vi "探头数据读取.vi"(11 "编号":string) -> ()   [LabVIEW 2016, in "斯坦道多参数.lvlib"]
panel:
  out "日期/时间字符串 2":string
  out "日期/时间字符串":string
  out "运行状态":u16(ring) items=["空闲", "水样测试", "标样核查"]
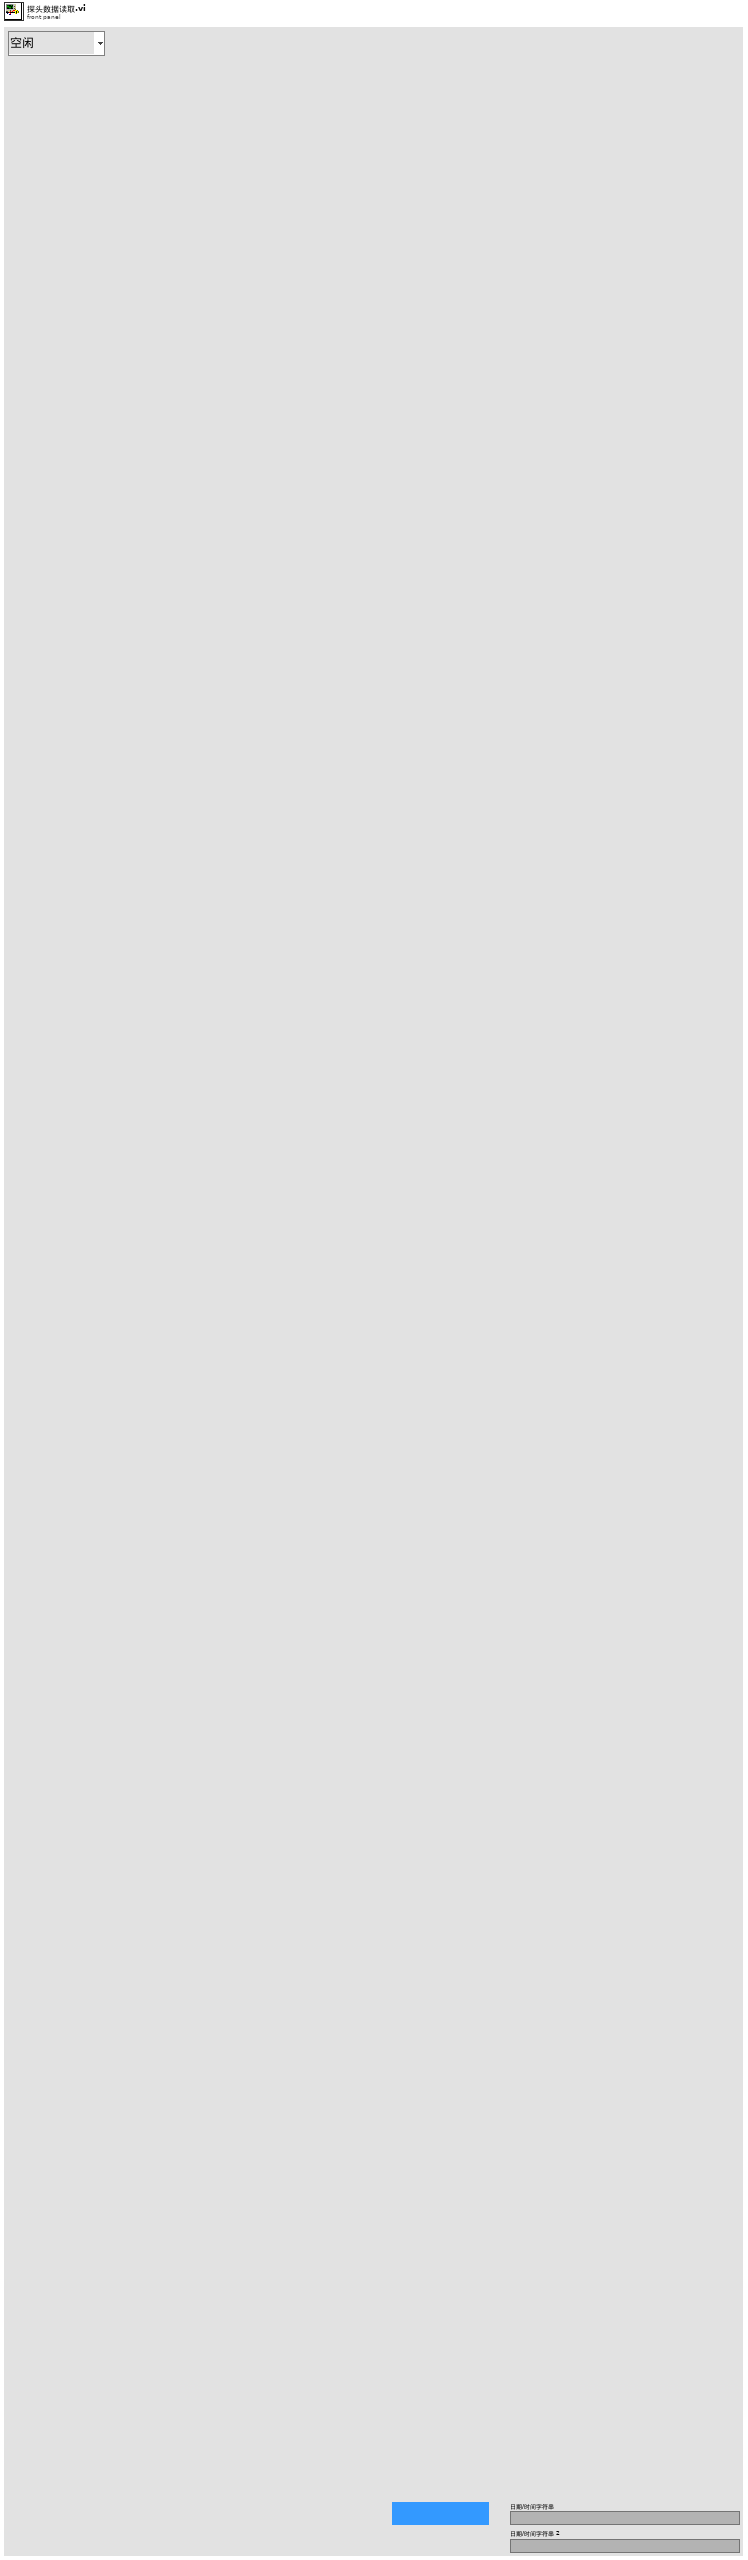
[diagram p1: front panel]
types:
  T1 = typedef "斯坦道多参数.lvlib/通知队列类型.ctl" = enum16{"pH", "DO", "DO2", "Cond", "Turb", "ORP", "叶绿素a", "藻密度", "COD"}
  T2 = cluster{"温度测量值":sgl, "测量值":sgl, "温度偏移修正值":sgl, "信号值":sgl, "数据标识":string}
  T3 = cluster{"温度测量值":sgl, "DO%":sgl, "DOmg/L":sgl, "温度偏移修正值":sgl, "数据标识mg/L":string, "数据标识%":string}
  T4 = cluster{"水温 (℃)":cluster{"量程下限":dbl, "量程上限":dbl}, "DO (mg/L)":cluster{"量程下限":dbl, "量程上限":dbl}, "DO (%)":cluster{"量程下限":dbl, "量程上限":dbl}, "pH":cluster{"量程下限":dbl, "量程上限":dbl}, "电导率 (μS/cm)":cluster{"量程下限":dbl, "量程上限":dbl}, "盐度":cluster{"量程下限":dbl, "量程上限":dbl}, "浊度 (NTU)":cluster{"量程下限":dbl, "量程上限":dbl}, "叶绿素a (μg/L)":cluster{"量程下限":dbl, "量程上限":dbl}, "藻密度 (cells/mL)":cluster{"量程下限":dbl, "量程上限":dbl}, "ORP (mV)":cluster{"量程下限":dbl, "量程上限":dbl}}
  T5 = cluster{"CH":u16, "监测值":dbl, "信号值":sgl, "数据标识":string}
  T6 = cluster{"pH探头选择":u16, "DO探头选择":u16, "电导率探头选择":u16, "浊度探头选择":u16, "叶绿素a探头选择":u16, "蓝绿藻探头选择":u16, "orp探头选择":u16, "COD探头选择":u16, "DO2探头选择":u16}
  T7 = cluster{"电极状态标志":u16, "电极型号标志":u16, "酸碱度测量值":sgl, "温度测量值":sgl, "酸碱度信号值":sgl, "温度信号值":sgl, "酸碱度偏移修正值":sgl, "温度偏移修正值":sgl, "手动温度补偿值":sgl, "酸碱度电极零点":sgl, "酸碱度电极斜率":sgl, "第1点标准值记录":sgl, "第1点信号值记录":sgl, "第1点温度值记录":sgl, "第2点标准值记录":sgl, "第2点信号值记录":sgl, "第2点温度值记录":sgl, "命令滤波设定":u16, "温度模式":enum16{"ATC", "MTC"}, "生产批次":u16, "电极序号":u16, "串口地址":u16, "串口波特率":enum16{"9600", "19200", "115200"}, "串口校验位":enum16{"NONE", "ODD", "EVEN"}, "串口停止位":enum16{"1bit", "2bit"}, "第一点标准值":sgl, "第二点标准值":sgl}
  T8 = cluster{"报警码":u16, "pH数值":sgl, "0X0003_NC":sgl, "温度数据":sgl, "pH原始信号 mv":sgl, "0X0009_NC":string, "产品名称":string, "序列号":string, "硬件版本":string, "软件版本":string, "通讯地址":u16, "波特率":u16, "设备类型":u16, "0X0026_NC":string, "第一点原始数据":sgl, "第一点校准数据":sgl, "第二点原始数据":sgl, "第二点校准数据":sgl, "探头校准命令":u16, "温度校准参数":sgl, "温度校准命令":u16}
  T9 = cluster{"电极状态标志":u16, "电极型号标志":u16, "电导率测量值":sgl, "温度测量值":sgl, "电导率信号值":sgl, "温度信号值":sgl, "温度补偿系数":sgl, "电导率偏移修正值":sgl, "温度偏移修正值":sgl, "手动温度补偿值":sgl, "电导率电极零点":sgl, "电导率电极斜率":sgl, "命令滤波设定":u16, "温度模式":enum16{"ATC", "MTC"}, "生产批次":u16, "电极序号":u16, "串口地址":u16, "串口波特率":enum16{"9600", "19200", "115200"}, "串口校验位":enum16{"NONE", "ODD", "EVEN"}, "串口停止位":enum16{"1bit", "2bit"}, "第一点标准值":sgl, "第二点标准值":sgl}
  T10 = cluster{"报警码":u16, "电导率数据（uS/cm）":sgl, "0x0003 NC":sgl, "温度数据":sgl, "电导率原始信号电阻":sgl, "当前量程":u16, "温度补偿系数":sgl, "0X0009_NC":string, "产品名称":string, "序列号":string, "硬件版本":string, "软件版本":string, "通讯地址":u16, "波特率":u16, "设备类型":u16, "0X0026_NC":string, "第一点原始数据":sgl, "第一点校准数据":sgl, "0X0035_NC":sgl, "0X0037_NC":sgl, "探头校准命令":u16, "温度校准参数":sgl, "温度校准命令":u16}
  T11 = cluster{"电极状态标志":u16, "电极型号标志":u16, "溶解氧测量值":sgl, "温度测量值":sgl, "溶解氧饱和度值":sgl, "盐度补偿值":sgl, "大气压补偿值":sgl, "溶解氧偏移修正值":sgl, "温度偏移修正值":sgl, "手动温度补偿值":sgl, "溶解氧电极零点":sgl, "溶解氧电极斜率":sgl, "第1点标准值记录":sgl, "第1点信号值记录":sgl, "第1点温度值记录":sgl, "第2点标准值记录":sgl, "第2点信号值记录":sgl, "第2点温度值记录":sgl, "命令滤波设定":u16, "温度模式":enum16{"ATC", "MTC"}, "生产批次":u16, "电极序号":u16, "串口地址":u16, "串口波特率":enum16{"9600", "19200", "115200"}, "串口校验位":enum16{"NONE", "ODD", "EVEN"}, "串口停止位":enum16{"1bit", "2bit"}, "第一点标准值":sgl, "第二点标准值":sgl}
  T12 = cluster{"报警码":u16, "溶解氧数值（mg/L）":sgl, "溶解氧数据（%）":sgl, "温度数据":sgl, "溶解氧原始信号 nA":sgl, "大气压力":sgl, "盐度":sgl, "0X0009_NC":string, "产品名称":string, "序列号":string, "硬件版本":string, "软件版本":string, "通讯地址":u16, "波特率":u16, "设备类型":u16, "0X0026_NC":string, "第一点原始数据":sgl, "0X0033 NC":sgl, "第二点原始数据":sgl, "0X0037 NC":sgl, "探头校准命令":u16, "温度校准参数":sgl, "温度校准命令":u16}
  T13 = cluster{"电极状态标志":u16, "电极型号标志":u16, "浊度测量值":sgl, "温度测量值":sgl, "浊度信号值":sgl, "浊度偏移修正值":sgl, "温度偏移修正值":sgl, "手动温度补偿值":sgl, "浊度电极零点":sgl, "浊度电极斜率":sgl, "清洁周期":u16, "命令滤波设定":u16, "温度模式":enum16{"ATC", "MTC"}, "生产批次":u16, "电极序号":u16, "串口地址":u16, "串口波特率":enum16{"9600", "19200", "115200"}, "串口校验位":enum16{"NONE", "ODD", "EVEN"}, "串口停止位":enum16{"1bit", "2bit"}, "第一点标准值":sgl, "第二点标准值":sgl, "第三点标准值":sgl}
  T14 = cluster{"报警码":u16, "浊度数值 NTU":sgl, "温度数据":sgl, "原始光强数值":u16, "量程":u16, "平均次数":u16, "清扫模式":u16, "清扫次数":u16, "清扫间隔分钟":u16, "0X000B_NC":string, "产品名称":string, "序列号":string, "硬件版本":string, "软件版本":string, "通讯地址":u16, "波特率":u16, "设备类型":u16, "0X0026_NC":string, "校准量程":u16, "第一点原始光强":u16, "第一点校准数据":sgl, "第二点原始光强":u16, "第二点校准数据":sgl, "第三点原始光强":u16, "第三点校准数据":sgl, "探头校准命令":u16, "温度校准参数":sgl, "温度校准命令":u16}
  T15 = cluster{"电极状态标志":u16, "电极型号标志":u16, "测量值":sgl, "温度测量值":sgl, "信号值":sgl, "温度信号值":sgl, "000AH_NC":sgl, "偏移修正值":sgl, "温度偏移修正值":sgl, "手动温度补偿值":sgl, "命令滤波设定":u16, "温度模式":enum16{"ATC", "MTC"}, "生产批次":u16, "传感器序号":u16, "串口地址":u16, "串口波特率":enum16{"9600", "19200", "115200"}, "串口校验位":enum16{"NONE", "ODD", "EVEN"}, "串口停止位":enum16{"1bit", "2bit"}}
  T16 = cluster{"报警码":u16, "叶绿素a":sgl, "温度数据":sgl, "原始光强数值":u16, "量程":u16, "平均次数":u16, "清扫模式":u16, "清扫次数":u16, "清扫间隔分钟":u16, "0X000B_NC":string, "产品名称":string, "序列号":string, "硬件版本":string, "软件版本":string, "通讯地址":u16, "波特率":u16, "设备类型":u16, "0X0026_NC":string, "校准量程":u16, "第一点原始光强":u16, "第一点校准数据":sgl, "第二点原始光强":u16, "第二点校准数据":sgl, "第三点原始光强":u16, "第三点校准数据":sgl, "探头校准命令":u16, "温度校准参数":sgl, "温度校准命令":u16}
  T17 = cluster{"报警码":u16, "蓝绿藻":sgl, "温度数据":sgl, "原始光强数值":u16, "0X0006_NC":u16, "平均次数":u16, "清扫模式":u16, "清扫次数":u16, "清扫间隔分钟":u16, "0X000B_NC":string, "产品名称":string, "序列号":string, "硬件版本":string, "软件版本":string, "通讯地址":u16, "波特率":u16, "设备类型":u16, "0X0026_NC":string, "0X0030_NC":u16, "第一点原始光强":u16, "第一点校准数据":sgl, "第二点原始光强":u16, "第二点校准数据":sgl, "第三点原始光强":u16, "第三点校准数据":sgl, "探头校准命令":u16, "温度校准参数":sgl, "温度校准命令":u16}
  T18 = cluster{"电极状态标志":u16, "电极型号标志":u16, "COD测量值":sgl, "浊度测量值":sgl, "COD信号值":sgl, "浊度信号值":sgl, "温度测量值":sgl, "COD偏移修正值":sgl, "浊度偏移修正值":sgl, "COD水样校正值":sgl, "温度偏移修正值":sgl, "COD零点系数":sgl, "COD斜率系数":sgl, "浊度零点系数":sgl, "浊度斜率系数":sgl, "COD测值K值":sgl, "浊度测值K值":sgl, "浊度补偿COD系数值":sgl, "COD温度补偿系数值 ":sgl, "测量周期":u16, "清洗周期":u16, "命令寄存器":u16, "数字滤波设定":u16, "温度模式":enum16{"AUTO", "OFF"}, "生产批次":u16, "电极序号":u16, "串口地址":u16, "串口波特率":enum16{"9600", "19200", "115200"}, "串口校验位":enum16{"NONE", "ODD", "EVEN"}, "串口停止位":enum16{"1bit", "2bit"}, "第一点校正指令":u16, "第一点标准值":sgl, "第二点校正指令":u16, "第二点标准值":sgl, "第三点校正指令":u16, "第三点标准值":sgl, "COD吸光度":sgl, "浊度吸光度":sgl, "温度信号值":sgl}
  T19 = cluster{"ph":bool, "DO":bool, "Cond":bool, "Turb":bool, "叶绿素a":bool, "藻密度":bool, "ORP":bool, "COD":bool, "DO2":bool}
  T20 = cluster{"ph":bool, "DO":bool, "Cond":bool, "Turb":bool, "叶绿素a":bool, "藻密度":bool, "ORP":bool, "cod":bool, "DO2":bool}
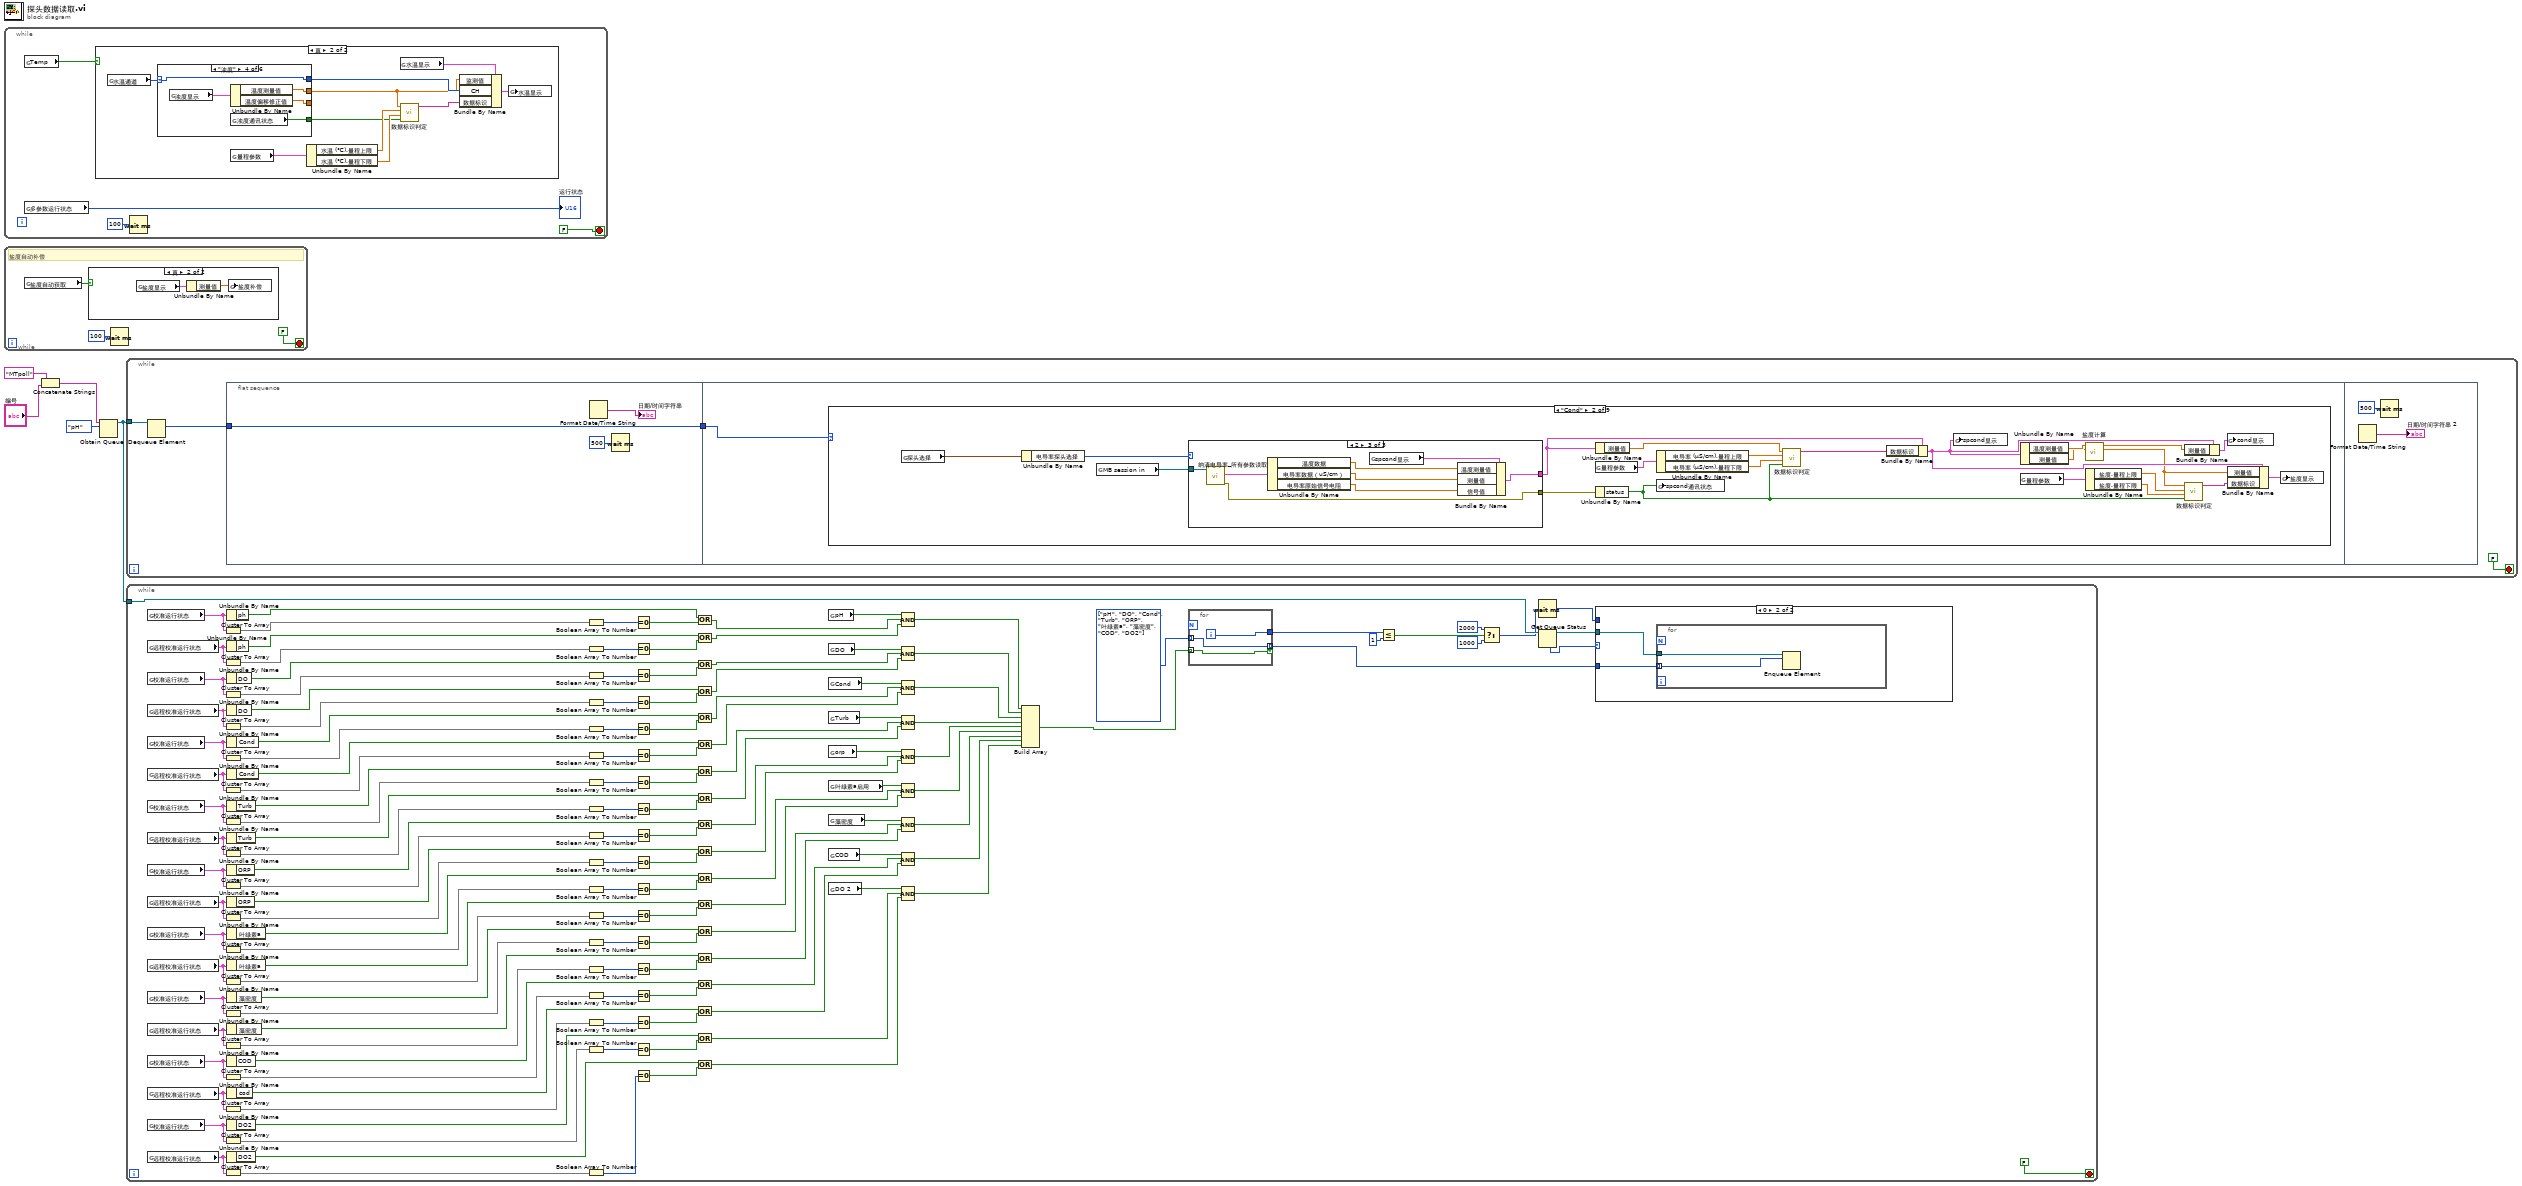
[diagram p0: block diagram]
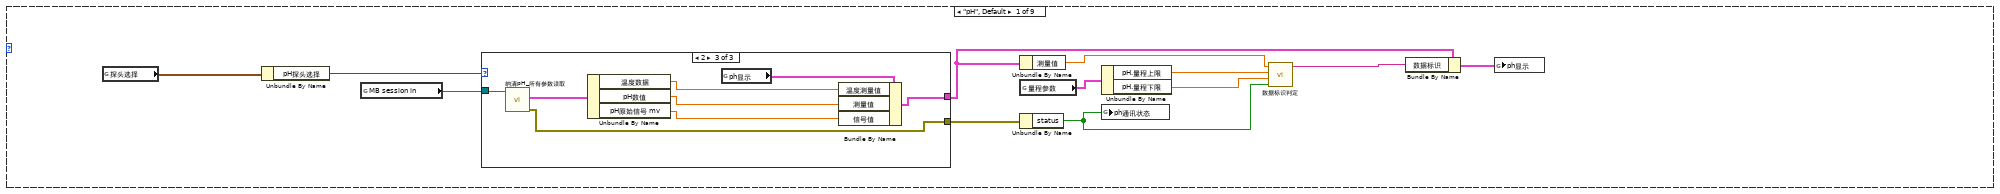
[diagram p3: hidden frame]
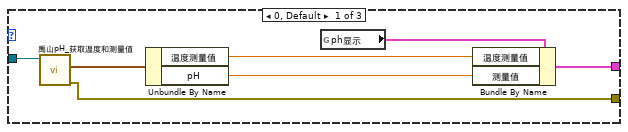
[diagram p4: hidden frame]
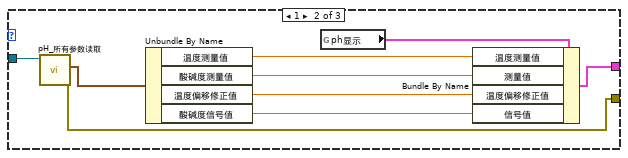
[diagram p5: hidden frame]
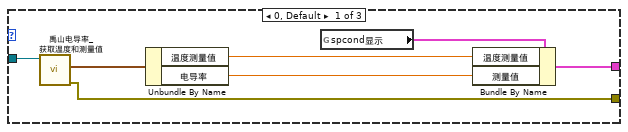
[diagram p6: hidden frame]
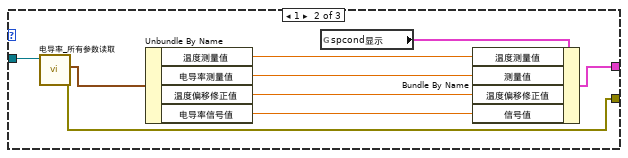
[diagram p7: hidden frame]
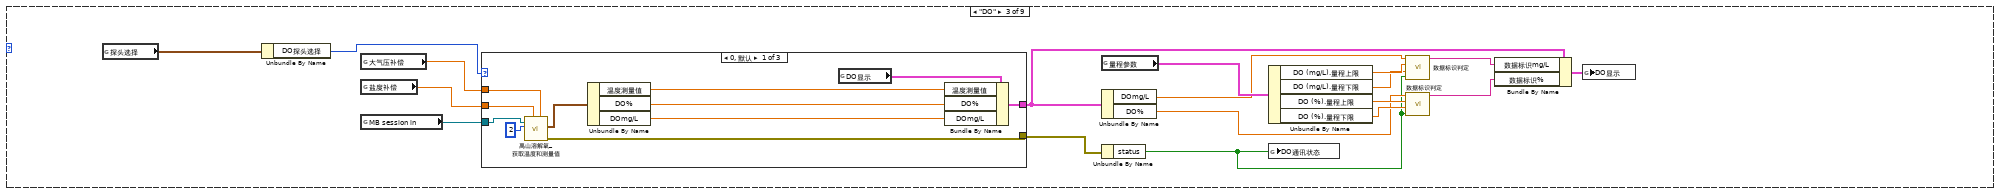
[diagram p8: hidden frame]
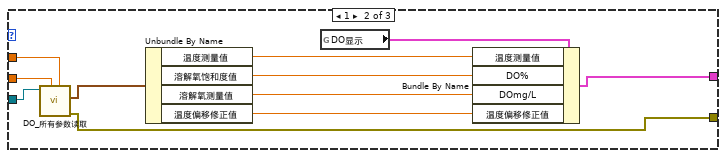
[diagram p9: hidden frame]
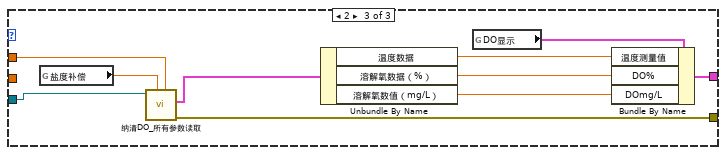
[diagram p10: hidden frame]
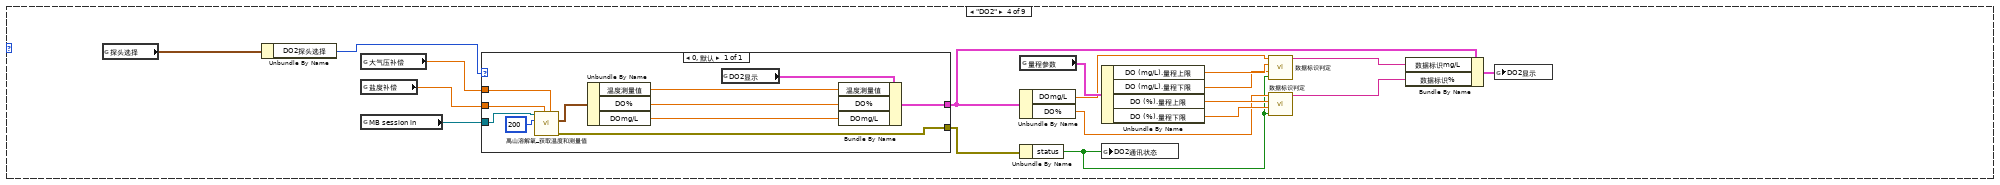
[diagram p11: hidden frame]
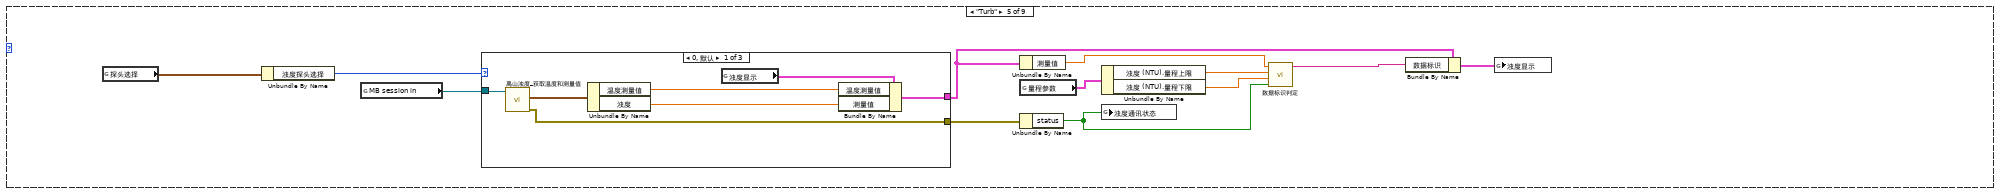
[diagram p12: hidden frame]
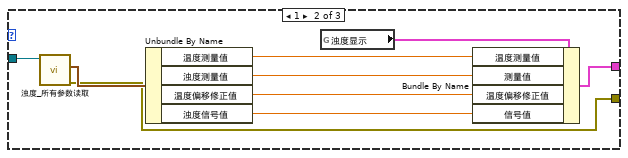
[diagram p13: hidden frame]
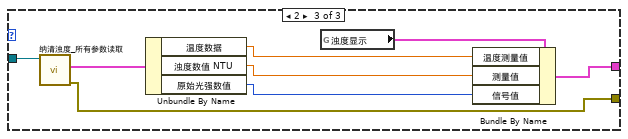
[diagram p14: hidden frame]
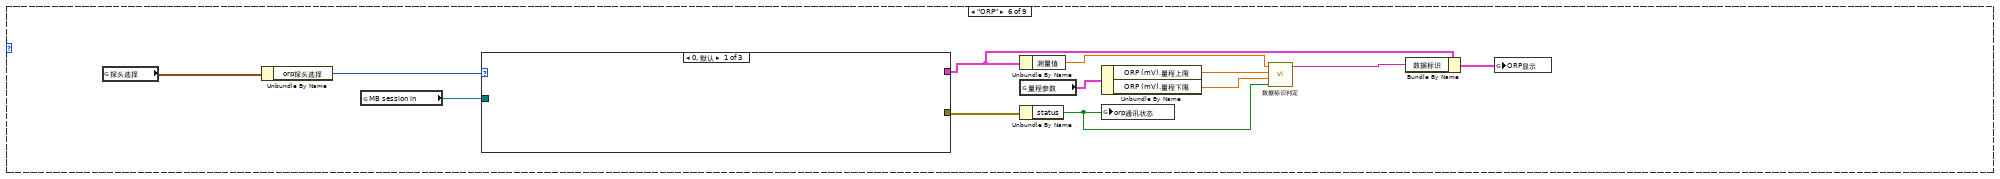
[diagram p15: hidden frame]
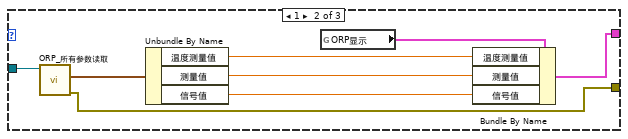
[diagram p16: hidden frame]
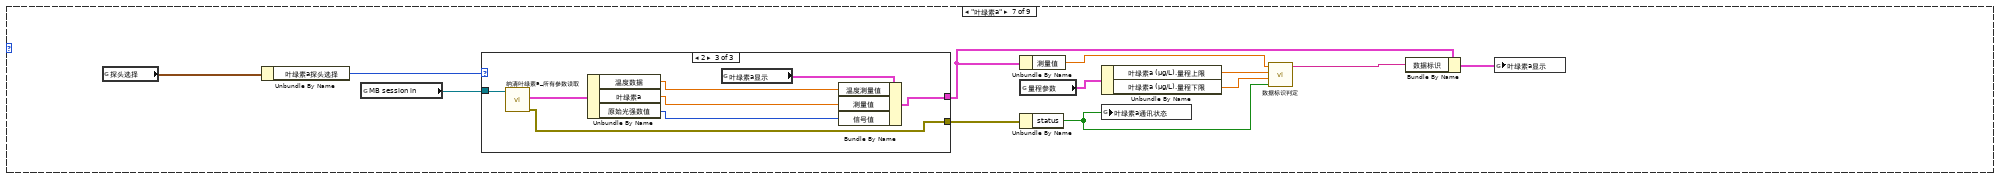
[diagram p18: hidden frame]
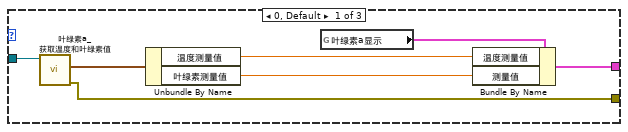
[diagram p19: hidden frame]
diagram:
  n1 = while {
    stop <- FALSE stop-if-true
    n2 = global read "断电保存变量.vi" "Temp"() -> (w7:bool)
    n3 = global read "多参数全局变量.vi" "多参数运行状态"() -> (→"运行状态":u16)
    n4 = case shown="真" w7 {
      frame False {
      }
      frame True {
        n5 = global read "断电保存变量.vi" "水温通道"() -> (w19:enum16{"pH", "DO", "浊度", "电导率", "叶绿素a", "藻密度"})
        n6 = case shown="\"浊度\"" w19 {
          selector: w19 -> [w24 w29 w34 w39 w44 w49]
          tunnel: [w24 w29 w34 w39 w44 w49] -> w18
          tunnel: [w22 w26 w31 w36 w41 w46] -> _
          tunnel: [w23 w27 w32 w37 w42 w47] -> w12
          tunnel: [w20 w25 w30 w35 w40 w45] -> w10
          frame "pH", Default {
            n7 = global read "多参数全局变量.vi" "ph显示"() -> (w21:T2)
            n8 = Unbundle By Name(w21) -> ("温度测量值"=w23:sgl, "温度偏移修正值"=w22:sgl)
            n9 = global read "多参数全局变量.vi" "ph通讯状态"() -> (w20:bool)
          }
          frame "电导率" {
            n10 = global read "多参数全局变量.vi" "spcond显示"() -> (w28:T2)
            n11 = Unbundle By Name(w28) -> ("温度测量值"=w27:sgl, "温度偏移修正值"=w26:sgl)
            n12 = global read "多参数全局变量.vi" "spcond通讯状态"() -> (w25:bool)
          }
          frame "DO" {
            n13 = global read "多参数全局变量.vi" "DO显示"() -> (w33:T3)
            n14 = Unbundle By Name(w33) -> ("温度测量值"=w32:sgl, "温度偏移修正值"=w31:sgl)
            n15 = global read "多参数全局变量.vi" "DO通讯状态"() -> (w30:bool)
          }
          frame "浊度" {
            n16 = global read "多参数全局变量.vi" "浊度显示"() -> (w38:T2)
            n17 = Unbundle By Name(w38) -> ("温度测量值"=w37:sgl, "温度偏移修正值"=w36:sgl)
            n18 = global read "多参数全局变量.vi" "浊度通讯状态"() -> (w35:bool)
          }
          frame "叶绿素a" {
            n19 = global read "多参数全局变量.vi" "叶绿素a显示"() -> (w43:T2)
            n20 = Unbundle By Name(w43) -> ("温度测量值"=w42:sgl, "温度偏移修正值"=w41:sgl)
            n21 = global read "多参数全局变量.vi" "叶绿素a通讯状态"() -> (w40:bool)
          }
          frame "藻密度" {
            n22 = global read "多参数全局变量.vi" "藻密度显示"() -> (w48:T2)
            n23 = Unbundle By Name(w48) -> ("温度测量值"=w47:sgl, "温度偏移修正值"=w46:sgl)
            n24 = global read "多参数全局变量.vi" "藻密度通讯状态"() -> (w45:bool)
          }
        }
        n25 = global read "断电保存变量.vi" "量程参数"() -> (w15:T4)
        n26 = Unbundle By Name(w15) -> ("水温 (℃).量程上限"=w13:dbl, "水温 (℃).量程下限"=w14:dbl)
        n27 = global read "多参数全局变量.vi" "水温显示"() -> (w16:T5)
        n28 = call "数据标识判定.vi"("通讯故障"=w10, "量程下限"=w14, "量程上限"=w13, "测量值"=w12) -> ("数据标识"=w11:string)  [unwired: 7 in]
        n29 = Bundle By Name(cluster=w16, "监测值"=w12, "CH"=w18, "数据标识"=w11) -> (w17:T5)
        n30 = global write "多参数全局变量.vi" "水温显示"(w17) -> ()
      }
    }
    n31 = Wait (ms)(milliseconds to wait=u32 100 ("等待时间（毫秒）")) -> ()  [unwired: 1 out]
  }
  n32 = while {
    stop <- FALSE stop-if-true
    # "盐度自动补偿"
    n33 = global read "断电保存变量.vi" "盐度自动获取"() -> (w51:bool)
    n34 = case shown="真" w51 {
      frame False {
      }
      frame True {
        n35 = global read "多参数全局变量.vi" "盐度显示"() -> (w54:T2)
        n36 = Unbundle By Name(w54) -> ("测量值"=w53:sgl)
        n37 = global write "断电保存变量.vi" "盐度补偿"(w53) -> ()
      }
    }
    n38 = Wait (ms)(milliseconds to wait=u32 100 ("等待时间（毫秒）")) -> ()  [unwired: 1 out]
  }
  n39 = Concatenate Strings("MTpoll" ("名称（未命名）"), "编号") -> (w3:string)
  n40 = Obtain Queue(name (unnamed)=w3, element data type=通知队列类型."pH" ("枚举")) -> (queue out=w1:refnum<queue>)  [unwired: 3 in, 2 out]
  n41 = while {
    tunnel: w1 -> [w58]
    stop <- FALSE stop-if-true
    n42 = Dequeue Element(queue=w58) -> (element=w57:T1)  [unwired: 2 in, 3 out]
    n43 = flat-sequence {
      tunnel: w57 -> [w61]
      tunnel: [w61] -> w55
      tunnel: w55 -> [w62]
      frame #0 {
        n44 = Format Date/Time String() -> (date/time string=→"日期/时间字符串":string)  [unwired: 3 in]
        n45 = Wait (ms)(milliseconds to wait=u32 500 ("等待时间（毫秒）")) -> ()  [unwired: 1 out]
      }
      frame #1 {
        n46 = case shown="\"Cond\"" w62 {
          frame "pH", Default {
            n47 = global read "断电保存变量.vi" "探头选择"() -> (w74:T6)
            n48 = Unbundle By Name(w74) -> ("pH探头选择"=w73:u16)
            n49 = global read "多参数全局变量.vi" "MB session in"() -> (w72:refnum<class "MB_Master.lvclass">)
            n50 = case shown="2" w73 {
              tunnel: w72 -> [w81 w90 w96]
              tunnel: [w80 w89 w94] -> w71
              tunnel: [w78 w86 w97] -> w70
              frame 0, Default {
                n51 = call "禹山pH_获取温度和测量值.vi"("MB session in"=w81) -> ("error out"=w80:errorcluster, "输出值"=w77:cluster{"温度测量值":sgl, "ORP":sgl, "pH":sgl})  [unwired: 8 in, 1 out]
                n52 = Unbundle By Name(w77) -> ("温度测量值"=w76:sgl, "pH"=w75:sgl)
                n53 = global read "多参数全局变量.vi" "ph显示"() -> (w79:T2)
                n54 = Bundle By Name(cluster=w79, "温度测量值"=w76, "测量值"=w75) -> (w78:T2)
              }
              frame 1 {
                n55 = call "pH_所有参数读取.vi"("MB session in"=w90) -> ("error out"=w89:errorcluster, "输出值"=w88:T7)  [unwired: 8 in, 1 out]
                n56 = Unbundle By Name(w88) -> ("温度测量值"=w83:sgl, "酸碱度测量值"=w84:sgl, "温度偏移修正值"=w85:sgl, "酸碱度信号值"=w82:sgl)
                n57 = global read "多参数全局变量.vi" "ph显示"() -> (w87:T2)
                n58 = Bundle By Name(cluster=w87, "温度测量值"=w83, "测量值"=w84, "温度偏移修正值"=w85, "信号值"=w82) -> (w86:T2)
              }
              frame 2 {
                n59 = call "纳清pH_所有参数读取.vi"("MB session in"=w96) -> ("error out"=w94:errorcluster, "输出值"=w95:T8)  [unwired: 8 in, 1 out]
                n60 = Unbundle By Name(w95) -> ("温度数据"=w93:sgl, "pH数值"=w92:sgl, "pH原始信号 mv"=w91:sgl)
                n61 = global read "多参数全局变量.vi" "ph显示"() -> (w98:T2)
                n62 = Bundle By Name(cluster=w98, "温度测量值"=w93, "测量值"=w92, "信号值"=w91) -> (w97:T2)
              }
            }
            n63 = Unbundle By Name(w70) -> ("测量值"=w68:sgl)
            n64 = global read "断电保存变量.vi" "量程参数"() -> (w69:T4)
            n65 = Unbundle By Name(w71) -> ("status"=w65:bool)
            n66 = Unbundle By Name(w69) -> ("pH.量程上限"=w67:dbl, "pH.量程下限"=w66:dbl)
            n67 = global write "多参数全局变量.vi" "ph通讯状态"(w65) -> ()
            n68 = call "数据标识判定.vi"("通讯故障"=w65, "量程下限"=w66, "量程上限"=w67, "测量值"=w68) -> ("数据标识"=w63:string)  [unwired: 7 in]
            n69 = Bundle By Name(cluster=w70, "数据标识"=w63) -> (w64:T2)
            n70 = global write "多参数全局变量.vi" "ph显示"(w64) -> ()
          }
          frame "Cond" {
            n71 = global read "断电保存变量.vi" "探头选择"() -> (w120:T6)
            n72 = Unbundle By Name(w120) -> ("电导率探头选择"=w119:u16)
            n73 = global read "多参数全局变量.vi" "MB session in"() -> (w118:refnum<class "MB_Master.lvclass">)
            n74 = case shown="2" w119 {
              tunnel: w118 -> [w127 w136 w140]
              tunnel: [w121 w134 w143] -> w113
              tunnel: [w126 w133 w138] -> w117
              frame 0, Default {
                n75 = call "禹山电导率_获取温度和测量值.vi"("MB session in"=w127) -> ("error out"=w126:errorcluster, "输出值"=w124:cluster{"温度测量值":sgl, "电导率":sgl, "错误标志":u16})  [unwired: 8 in, 1 out]
                n76 = Unbundle By Name(w124) -> ("温度测量值"=w123:sgl, "电导率"=w122:sgl)
                n77 = global read "多参数全局变量.vi" "spcond显示"() -> (w125:T2)
                n78 = Bundle By Name(cluster=w125, "温度测量值"=w123, "测量值"=w122) -> (w121:T2)
              }
              frame 1 {
                n79 = call "电导率_所有参数读取.vi"("MB session in"=w136) -> ("error out"=w133:errorcluster, "输出值"=w132:T9)  [unwired: 8 in, 1 out]
                n80 = Unbundle By Name(w132) -> ("温度测量值"=w131:sgl, "电导率测量值"=w130:sgl, "温度偏移修正值"=w129:sgl, "电导率信号值"=w128:sgl)
                n81 = global read "多参数全局变量.vi" "spcond显示"() -> (w135:T2)
                n82 = Bundle By Name(cluster=w135, "温度测量值"=w131, "测量值"=w130, "温度偏移修正值"=w129, "信号值"=w128) -> (w134:T2)
              }
              frame 2 {
                n83 = call "纳清电导率_所有参数读取.vi"("MB session in"=w140) -> ("error out"=w138:errorcluster, "输出值"=w139:T10)  [unwired: 8 in, 1 out]
                n84 = Unbundle By Name(w139) -> ("温度数据"=w142:sgl, "电导率数据（uS/cm）"=w141:sgl, "电导率原始信号电阻"=w137:sgl)
                n85 = global read "多参数全局变量.vi" "spcond显示"() -> (w144:T2)
                n86 = Bundle By Name(cluster=w144, "温度测量值"=w142, "测量值"=w141, "信号值"=w137) -> (w143:T2)
              }
            }
            n87 = Unbundle By Name(w113) -> ("测量值"=w112:sgl)
            n88 = global read "断电保存变量.vi" "量程参数"() -> (w116:T4)
            n89 = Unbundle By Name(w117) -> ("status"=w109:bool)
            n90 = Unbundle By Name(w116) -> ("电导率 (μS/cm).量程上限"=w115:dbl, "电导率 (μS/cm).量程下限"=w114:dbl)
            n91 = global write "多参数全局变量.vi" "spcond通讯状态"(w109) -> ()
            n92 = call "数据标识判定.vi"("通讯故障"=w109, "量程下限"=w114, "量程上限"=w115, "测量值"=w112) -> ("数据标识"=w110:string)  [unwired: 7 in]
            n93 = Bundle By Name(cluster=w113, "数据标识"=w110) -> (w111:T2)
            n94 = global write "多参数全局变量.vi" "spcond显示"(w111) -> ()
            n95 = Unbundle By Name(w111) -> ("温度测量值"=w108:sgl, "测量值"=w107:sgl)
            n96 = global read "断电保存变量.vi" "量程参数"() -> (w101:T4)
            n97 = call "盐度计算.vi"("spCond"=w107, "Temp"=w108) -> ("saltresult"=w100:dbl, "cond"=w106:dbl)  [unwired: 8 in]
            n98 = Unbundle By Name(w101) -> ("盐度.量程上限"=w102:dbl, "盐度.量程下限"=w103:dbl)
            n99 = Bundle By Name(cluster=w111, "测量值"=w106) -> (w105:T2)
            n100 = call "数据标识判定.vi"("通讯故障"=w109, "量程下限"=w103, "量程上限"=w102, "测量值"=w100) -> ("数据标识"=w99:string)  [unwired: 7 in]
            n101 = global write "多参数全局变量.vi" "cond显示"(w105) -> ()
            n102 = Bundle By Name(cluster=w111, "测量值"=w100, "数据标识"=w99) -> (w104:T2)
            n103 = global write "多参数全局变量.vi" "盐度显示"(w104) -> ()
          }
          frame "DO" {
            n104 = global read "断电保存变量.vi" "探头选择"() -> (w162:T6)
            n105 = Unbundle By Name(w162) -> ("DO探头选择"=w161:u16)
            n106 = global read "断电保存变量.vi" "大气压补偿"() -> (w145:dbl)
            n107 = global read "断电保存变量.vi" "盐度补偿"() -> (w146:dbl)
            n108 = global read "多参数全局变量.vi" "MB session in"() -> (w160:refnum<class "MB_Master.lvclass">)
            n109 = case shown="0, 默认" w161 {
              tunnel: w160 -> [w173 w184 w189]
              tunnel: [w171 w182 w193] -> w153
              tunnel: [w167 w177 w187] -> w159
              tunnel: w146 -> [w164 w175 _]
              tunnel: w145 -> [w163 w174 w185]
              frame 0, Default {
                n110 = call "禹山溶解氧_获取温度和测量值.vi"("大气压补偿"=w163, "盐度补偿"=w164, "salve ID"=u16 2, "MB session in"=w173) -> ("error out"=w167:errorcluster, "输出值"=w166:cluster{"温度测量值":sgl, "DO%":sgl, "DOmg/L":sgl})  [unwired: 5 in, 1 out]
                n111 = Unbundle By Name(w166) -> ("温度测量值"=w170:sgl, "DO%"=w169:sgl, "DOmg/L"=w168:sgl)
                n112 = global read "多参数全局变量.vi" "DO显示"() -> (w172:T3)
                n113 = Bundle By Name(cluster=w172, "温度测量值"=w170, "DO%"=w169, "DOmg/L"=w168) -> (w171:T3)
              }
              frame 1 {
                n114 = call "DO_所有参数读取.vi"("大气压补偿"=w174, "盐度补偿"=w175, "MB session in"=w184) -> ("error out"=w177:errorcluster, "输出值"=w181:T11)  [unwired: 6 in, 1 out]
                n115 = Unbundle By Name(w181) -> ("温度测量值"=w178:sgl, "溶解氧饱和度值"=w179:sgl, "溶解氧测量值"=w180:sgl, "温度偏移修正值"=w176:sgl)
                n116 = global read "多参数全局变量.vi" "DO显示"() -> (w183:T3)
                n117 = Bundle By Name(cluster=w183, "温度测量值"=w178, "DO%"=w179, "DOmg/L"=w180, "温度偏移修正值"=w176) -> (w182:T3)
              }
              frame 2 {
                n118 = global read "断电保存变量.vi" "盐度补偿"() -> (w186:dbl)
                n119 = call "纳清DO_所有参数读取.vi"("大气压补偿"=w185, "盐度补偿"=w186, "MB session in"=w189) -> ("error out"=w187:errorcluster, "输出值"=w188:T12)  [unwired: 6 in, 1 out]
                n120 = Unbundle By Name(w188) -> ("温度数据"=w190:sgl, "溶解氧数据（%）"=w191:sgl, "溶解氧数值（mg/L）"=w192:sgl)
                n121 = global read "多参数全局变量.vi" "DO显示"() -> (w194:T3)
                n122 = Bundle By Name(cluster=w194, "温度测量值"=w190, "DO%"=w191, "DOmg/L"=w192) -> (w193:T3)
              }
            }
            n123 = global read "断电保存变量.vi" "量程参数"() -> (w158:T4)
            n124 = Unbundle By Name(w153) -> ("DOmg/L"=w152:sgl, "DO%"=w151:sgl)
            n125 = Unbundle By Name(w159) -> ("status"=w147:bool)
            n126 = Unbundle By Name(w158) -> ("DO (mg/L).量程上限"=w157:dbl, "DO (mg/L).量程下限"=w156:dbl, "DO (%).量程上限"=w155:dbl, "DO (%).量程下限"=w154:dbl)
            n127 = global write "多参数全局变量.vi" "DO通讯状态"(w147) -> ()
            n128 = call "数据标识判定.vi"("通讯故障"=w147, "量程下限"=w156, "量程上限"=w157, "测量值"=w152) -> ("数据标识"=w149:string)  [unwired: 7 in]
            n129 = call "数据标识判定.vi"("通讯故障"=w147, "量程下限"=w154, "量程上限"=w155, "测量值"=w151) -> ("数据标识"=w148:string)  [unwired: 7 in]
            n130 = Bundle By Name(cluster=w153, "数据标识mg/L"=w149, "数据标识%"=w148) -> (w150:T3)
            n131 = global write "多参数全局变量.vi" "DO显示"(w150) -> ()
          }
          frame "DO2" {
            n132 = global read "断电保存变量.vi" "探头选择"() -> (w212:T6)
            n133 = Unbundle By Name(w212) -> ("DO2探头选择"=w211:u16)
            n134 = global read "断电保存变量.vi" "大气压补偿"() -> (w195:dbl)
            n135 = global read "断电保存变量.vi" "盐度补偿"() -> (w196:dbl)
            n136 = global read "多参数全局变量.vi" "MB session in"() -> (w210:refnum<class "MB_Master.lvclass">)
            n137 = case shown="0, 默认" w211 {
              tunnel: w210 -> [w223]
              tunnel: [w221] -> w203
              tunnel: [w217] -> w209
              tunnel: w196 -> [w214]
              tunnel: w195 -> [w213]
              frame 0, Default {
                n138 = call "禹山溶解氧_获取温度和测量值.vi"("大气压补偿"=w213, "盐度补偿"=w214, "salve ID"=u16 200, "MB session in"=w223) -> ("error out"=w217:errorcluster, "输出值"=w216:cluster{"温度测量值":sgl, "DO%":sgl, "DOmg/L":sgl})  [unwired: 5 in, 1 out]
                n139 = Unbundle By Name(w216) -> ("温度测量值"=w220:sgl, "DO%"=w219:sgl, "DOmg/L"=w218:sgl)
                n140 = global read "多参数全局变量.vi" "DO2显示"() -> (w222:T3)
                n141 = Bundle By Name(cluster=w222, "温度测量值"=w220, "DO%"=w219, "DOmg/L"=w218) -> (w221:T3)
              }
            }
            n142 = global read "断电保存变量.vi" "量程参数"() -> (w208:T4)
            n143 = Unbundle By Name(w203) -> ("DOmg/L"=w202:sgl, "DO%"=w201:sgl)
            n144 = Unbundle By Name(w209) -> ("status"=w197:bool)
            n145 = Unbundle By Name(w208) -> ("DO (mg/L).量程上限"=w207:dbl, "DO (mg/L).量程下限"=w206:dbl, "DO (%).量程上限"=w205:dbl, "DO (%).量程下限"=w204:dbl)
            n146 = global write "多参数全局变量.vi" "DO2通讯状态"(w197) -> ()
            n147 = call "数据标识判定.vi"("通讯故障"=w197, "量程下限"=w206, "量程上限"=w207, "测量值"=w202) -> ("数据标识"=w199:string)  [unwired: 7 in]
            n148 = call "数据标识判定.vi"("通讯故障"=w197, "量程下限"=w204, "量程上限"=w205, "测量值"=w201) -> ("数据标识"=w198:string)  [unwired: 7 in]
            n149 = Bundle By Name(cluster=w203, "数据标识mg/L"=w199, "数据标识%"=w198) -> (w200:T3)
            n150 = global write "多参数全局变量.vi" "DO2显示"(w200) -> ()
          }
          frame "Turb" {
            n151 = global read "断电保存变量.vi" "探头选择"() -> (w235:T6)
            n152 = Unbundle By Name(w235) -> ("浊度探头选择"=w234:u16)
            n153 = global read "多参数全局变量.vi" "MB session in"() -> (w233:refnum<class "MB_Master.lvclass">)
            n154 = case shown="0, 默认" w234 {
              tunnel: w233 -> [w242 w251 w255]
              tunnel: [w240 w246 w256] -> w227
              tunnel: [w239 w245 w254] -> w232
              frame 0, Default {
                n155 = call "禹山浊度_获取温度和测量值.vi"("MB session in"=w242) -> ("error out"=w239:errorcluster, "输出值"=w238:cluster{"温度测量值":sgl, "浊度":sgl})  [unwired: 8 in, 1 out]
                n156 = Unbundle By Name(w238) -> ("温度测量值"=w237:sgl, "浊度"=w236:sgl)
                n157 = global read "多参数全局变量.vi" "浊度显示"() -> (w241:T2)
                n158 = Bundle By Name(cluster=w241, "温度测量值"=w237, "测量值"=w236) -> (w240:T2)
              }
              frame 1 {
                n159 = call "浊度_所有参数读取.vi"("MB session in"=w251) -> ("error out"=w245:errorcluster, "输出值"=w250:T13)  [unwired: 8 in, 1 out]
                n160 = Unbundle By Name(w250) -> ("温度测量值"=w248:sgl, "浊度测量值"=w247:sgl, "温度偏移修正值"=w244:sgl, "浊度信号值"=w243:sgl)
                n161 = global read "多参数全局变量.vi" "浊度显示"() -> (w249:T2)
                n162 = Bundle By Name(cluster=w249, "温度测量值"=w248, "测量值"=w247, "温度偏移修正值"=w244, "信号值"=w243) -> (w246:T2)
              }
              frame 2 {
                n163 = call "纳清浊度_所有参数读取.vi"("MB session in"=w255) -> ("error out"=w254:errorcluster, "输出值"=w253:T14)  [unwired: 8 in, 1 out]
                n164 = Unbundle By Name(w253) -> ("温度数据"=w258:sgl, "浊度数值 NTU"=w257:sgl, "原始光强数值"=w252:u16)
                n165 = global read "多参数全局变量.vi" "浊度显示"() -> (w259:T2)
                n166 = Bundle By Name(cluster=w259, "温度测量值"=w258, "测量值"=w257, "信号值"=w252) -> (w256:T2)
              }
            }
            n167 = Unbundle By Name(w227) -> ("测量值"=w226:sgl)
            n168 = global read "断电保存变量.vi" "量程参数"() -> (w231:T4)
            n169 = Unbundle By Name(w232) -> ("status"=w228:bool)
            n170 = Unbundle By Name(w231) -> ("浊度 (NTU).量程上限"=w230:dbl, "浊度 (NTU).量程下限"=w229:dbl)
            n171 = global write "多参数全局变量.vi" "浊度通讯状态"(w228) -> ()
            n172 = call "数据标识判定.vi"("通讯故障"=w228, "量程下限"=w229, "量程上限"=w230, "测量值"=w226) -> ("数据标识"=w224:string)  [unwired: 7 in]
            n173 = Bundle By Name(cluster=w227, "数据标识"=w224) -> (w225:T2)
            n174 = global write "多参数全局变量.vi" "浊度显示"(w225) -> ()
          }
          frame "ORP" {
            n175 = global read "断电保存变量.vi" "探头选择"() -> (w271:T6)
            n176 = Unbundle By Name(w271) -> ("orp探头选择"=w270:u16)
            n177 = global read "多参数全局变量.vi" "MB session in"() -> (w269:refnum<class "MB_Master.lvclass">)
            n178 = case shown="0, 默认" w270 {
              tunnel: [_ w274 _] -> w268
              tunnel: w269 -> [_ w279 _]
              tunnel: [_ w272 _] -> w263
              frame 0, Default {
              }
              frame 1 {
                n179 = call "ORP_所有参数读取.vi"("MB session in"=w279) -> ("error out"=w274:errorcluster, "输出值"=w276:T15)  [unwired: 8 in, 1 out]
                n180 = Unbundle By Name(w276) -> ("温度测量值"=w277:sgl, "测量值"=w278:sgl, "信号值"=w273:sgl)
                n181 = global read "多参数全局变量.vi" "ORP显示"() -> (w275:T2)
                n182 = Bundle By Name(cluster=w275, "温度测量值"=w277, "测量值"=w278, "信号值"=w273) -> (w272:T2)
              }
              frame 2 {
              }
            }
            n183 = Unbundle By Name(w263) -> ("测量值"=w262:sgl)
            n184 = global read "断电保存变量.vi" "量程参数"() -> (w267:T4)
            n185 = Unbundle By Name(w268) -> ("status"=w264:bool)
            n186 = Unbundle By Name(w267) -> ("ORP (mV).量程上限"=w266:dbl, "ORP (mV).量程下限"=w265:dbl)
            n187 = global write "多参数全局变量.vi" "orp通讯状态"(w264) -> ()
            n188 = call "数据标识判定.vi"("通讯故障"=w264, "量程下限"=w265, "量程上限"=w266, "测量值"=w262) -> ("数据标识"=w260:string)  [unwired: 7 in]
            n189 = Bundle By Name(cluster=w263, "数据标识"=w260) -> (w261:T2)
            n190 = global write "多参数全局变量.vi" "ORP显示"(w261) -> ()
          }
          frame "叶绿素a" {
            n191 = global read "断电保存变量.vi" "探头选择"() -> (w291:T6)
            n192 = Unbundle By Name(w291) -> ("叶绿素a探头选择"=w290:u16)
            n193 = global read "多参数全局变量.vi" "MB session in"() -> (w289:refnum<class "MB_Master.lvclass">)
            n194 = case shown="2" w290 {
              tunnel: [w298 _ w304] -> w288
              tunnel: w289 -> [w297 _ w306]
              tunnel: [w295 _ w303] -> w284
              frame 0, Default {
                n195 = call "叶绿素a_获取温度和叶绿素值.vi"("MB session in"=w297) -> ("error out"=w298:errorcluster, "输出值"=w294:cluster{"温度测量值":sgl, "叶绿素测量值":sgl, "错误标志":u16})  [unwired: 8 in, 1 out]
                n196 = Unbundle By Name(w294) -> ("温度测量值"=w292:sgl, "叶绿素测量值"=w293:sgl)
                n197 = global read "多参数全局变量.vi" "叶绿素a显示"() -> (w296:T2)
                n198 = Bundle By Name(cluster=w296, "温度测量值"=w292, "测量值"=w293) -> (w295:T2)
              }
              frame 1 {
              }
              frame 2 {
                n199 = call "纳清叶绿素a_所有参数读取.vi"("MB session in"=w306) -> ("error out"=w304:errorcluster, "输出值"=w302:T16)  [unwired: 8 in, 1 out]
                n200 = Unbundle By Name(w302) -> ("温度数据"=w300:sgl, "叶绿素a"=w301:sgl, "原始光强数值"=w299:u16)
                n201 = global read "多参数全局变量.vi" "叶绿素a显示"() -> (w305:T2)
                n202 = Bundle By Name(cluster=w305, "温度测量值"=w300, "测量值"=w301, "信号值"=w299) -> (w303:T2)
              }
            }
            n203 = Unbundle By Name(w284) -> ("测量值"=w283:sgl)
            n204 = global read "断电保存变量.vi" "量程参数"() -> (w287:T4)
            n205 = Unbundle By Name(w288) -> ("status"=w282:bool)
            n206 = Unbundle By Name(w287) -> ("叶绿素a (μg/L).量程上限"=w286:dbl, "叶绿素a (μg/L).量程下限"=w285:dbl)
            n207 = global write "多参数全局变量.vi" "叶绿素a通讯状态"(w282) -> ()
            n208 = call "数据标识判定.vi"("通讯故障"=w282, "量程下限"=w285, "量程上限"=w286, "测量值"=w283) -> ("数据标识"=w280:string)  [unwired: 7 in]
            n209 = Bundle By Name(cluster=w284, "数据标识"=w280) -> (w281:T2)
            n210 = global write "多参数全局变量.vi" "叶绿素a显示"(w281) -> ()
          }
          frame "藻密度" {
            n211 = global read "断电保存变量.vi" "探头选择"() -> (w318:T6)
            n212 = Unbundle By Name(w318) -> ("蓝绿藻探头选择"=w317:u16)
            n213 = global read "多参数全局变量.vi" "MB session in"() -> (w316:refnum<class "MB_Master.lvclass">)
            n214 = case shown="2" w317 {
              tunnel: [_ _ w324] -> w315
              tunnel: w316 -> [_ _ w326]
              tunnel: [_ _ w323] -> w311
              frame 0, Default {
              }
              frame 1 {
              }
              frame 2 {
                n215 = call "纳清蓝绿藻_所有参数读取.vi"("MB session in"=w326) -> ("error out"=w324:errorcluster, "输出值"=w322:T17)  [unwired: 8 in, 1 out]
                n216 = Unbundle By Name(w322) -> ("温度数据"=w321:sgl, "蓝绿藻"=w320:sgl, "原始光强数值"=w319:u16)
                n217 = global read "多参数全局变量.vi" "藻密度显示"() -> (w325:T2)
                n218 = Bundle By Name(cluster=w325, "温度测量值"=w321, "测量值"=w320, "信号值"=w319) -> (w323:T2)
              }
            }
            n219 = Unbundle By Name(w311) -> ("测量值"=w310:sgl)
            n220 = global read "断电保存变量.vi" "量程参数"() -> (w314:T4)
            n221 = Unbundle By Name(w315) -> ("status"=w309:bool)
            n222 = Unbundle By Name(w314) -> ("藻密度 (cells/mL).量程上限"=w313:dbl, "藻密度 (cells/mL).量程下限"=w312:dbl)
            n223 = global write "多参数全局变量.vi" "藻密度通讯状态"(w309) -> ()
            n224 = call "数据标识判定.vi"("通讯故障"=w309, "量程下限"=w312, "量程上限"=w313, "测量值"=w310) -> ("数据标识"=w307:string)  [unwired: 7 in]
            n225 = Bundle By Name(cluster=w311, "数据标识"=w307) -> (w308:T2)
            n226 = global write "多参数全局变量.vi" "藻密度显示"(w308) -> ()
          }
          frame "COD" {
            n227 = global read "断电保存变量.vi" "探头选择"() -> (w337:T6)
            n228 = Unbundle By Name(w337) -> ("COD探头选择"=w336:u16)
            n229 = global read "多参数全局变量.vi" "MB session in"() -> (w335:refnum<class "MB_Master.lvclass">)
            n230 = case shown="1" w336 {
              tunnel: [_ w343 _] -> w334
              tunnel: w335 -> [_ w345 _]
              tunnel: [_ w342 _] -> w333
              frame 0, Default {
              }
              frame 1 {
                n231 = call "COD_所有参数读取.vi"("MB session in"=w345) -> ("error out"=w343:errorcluster, "输出值"=w341:T18)  [unwired: 8 in, 1 out]
                n232 = Unbundle By Name(w341) -> ("温度测量值"=w340:sgl, "COD测量值"=w339:sgl, "COD信号值"=w338:sgl)
                n233 = global read "多参数全局变量.vi" "COD显示"() -> (w344:T2)
                n234 = Bundle By Name(cluster=w344, "温度测量值"=w340, "测量值"=w339, "信号值"=w338) -> (w342:T2)
              }
              frame 2 {
              }
            }
            n235 = Unbundle By Name(w333) -> ("测量值"=w332:sgl)
            n236 = Unbundle By Name(w334) -> ("status"=w331:bool)
            n237 = global write "多参数全局变量.vi" "cod通讯状态"(w331) -> ()
            n238 = call "数据标识判定.vi"("通讯故障"=w331, "量程下限"=0.0, "量程上限"=1000.0, "测量值"=w332) -> ("数据标识"=w329:string)  [unwired: 7 in]
            n239 = Bundle By Name(cluster=w333, "数据标识"=w329) -> (w330:T2)
            n240 = case shown="无错误" w334 {
              tunnel: w330 -> [w346 _]
              frame No Error {
                n241 = global write "多参数全局变量.vi" "COD显示"(w346) -> ()
              }
              frame Error {
              }
            }
          }
        }
      }
      frame #2 {
        n242 = Format Date/Time String() -> (date/time string=→"日期/时间字符串 2":string)  [unwired: 3 in]
        n243 = Wait (ms)(milliseconds to wait=u32 500 ("等待时间（毫秒）")) -> ()  [unwired: 1 out]
      }
    }
  }
  n244 = while {
    tunnel: w1 -> [w488]
    stop <- FALSE stop-if-true
    w388 = T1[] [enum."pH", enum."DO", enum."Cond", enum."Turb", enum."ORP", enum."叶绿素a", enum."藻密度", enum."COD", enum."DO2"] items=["pH", "DO", "DO2", "Cond", "Turb", "ORP", "叶绿素a", "藻密度", "COD"]
    n245 = global read "多参数全局变量.vi" "校准运行状态"() -> (w474:T19)
    n246 = global read "多参数全局变量.vi" "远程校准运行状态"() -> (w485:T20)
    n247 = global read "多参数全局变量.vi" "校准运行状态"() -> (w448:T19)
    n248 = global read "多参数全局变量.vi" "远程校准运行状态"() -> (w459:T20)
    n249 = global read "多参数全局变量.vi" "校准运行状态"() -> (w473:T19)
    n250 = global read "多参数全局变量.vi" "远程校准运行状态"() -> (w462:T20)
    n251 = global read "多参数全局变量.vi" "校准运行状态"() -> (w435:T19)
    n252 = global read "多参数全局变量.vi" "远程校准运行状态"() -> (w446:T20)
    n253 = global read "多参数全局变量.vi" "校准运行状态"() -> (w422:T19)
    n254 = global read "多参数全局变量.vi" "远程校准运行状态"() -> (w433:T20)
    n255 = global read "多参数全局变量.vi" "校准运行状态"() -> (w421:T19)
    n256 = global read "多参数全局变量.vi" "远程校准运行状态"() -> (w410:T20)
    n257 = global read "多参数全局变量.vi" "校准运行状态"() -> (w396:T19)
    n258 = global read "多参数全局变量.vi" "远程校准运行状态"() -> (w407:T20)
    n259 = global read "多参数全局变量.vi" "校准运行状态"() -> (w383:T19)
    n260 = global read "多参数全局变量.vi" "远程校准运行状态"() -> (w376:T20)
    n261 = global read "多参数全局变量.vi" "校准运行状态"() -> (w369:T19)
    n262 = global read "多参数全局变量.vi" "远程校准运行状态"() -> (w358:T20)
    n263 = Cluster To Array(cluster=w474) -> (array=w479:bool[])
    n264 = Cluster To Array(cluster=w485) -> (array=w481:bool[])
    n265 = Cluster To Array(cluster=w448) -> (array=w453:bool[])
    n266 = Cluster To Array(cluster=w459) -> (array=w455:bool[])
    n267 = Cluster To Array(cluster=w473) -> (array=w468:bool[])
    n268 = Cluster To Array(cluster=w462) -> (array=w466:bool[])
    n269 = Cluster To Array(cluster=w435) -> (array=w440:bool[])
    n270 = Cluster To Array(cluster=w446) -> (array=w442:bool[])
    n271 = Cluster To Array(cluster=w422) -> (array=w427:bool[])
    n272 = Cluster To Array(cluster=w433) -> (array=w429:bool[])
    n273 = Cluster To Array(cluster=w421) -> (array=w416:bool[])
    n274 = Cluster To Array(cluster=w410) -> (array=w414:bool[])
    n275 = Cluster To Array(cluster=w396) -> (array=w401:bool[])
    n276 = Cluster To Array(cluster=w407) -> (array=w403:bool[])
    n277 = Cluster To Array(cluster=w383) -> (array=w379:bool[])
    n278 = Cluster To Array(cluster=w376) -> (array=w375:bool[])
    n279 = Cluster To Array(cluster=w369) -> (array=w364:bool[])
    n280 = Cluster To Array(cluster=w358) -> (array=w362:bool[])
    n281 = Unbundle By Name(w474) -> ("ph"=w476:bool)
    n282 = Unbundle By Name(w485) -> ("ph"=w484:bool)
    n283 = Unbundle By Name(w448) -> ("DO"=w450:bool)
    n284 = Unbundle By Name(w459) -> ("DO"=w458:bool)
    n285 = Unbundle By Name(w473) -> ("Cond"=w471:bool)
    n286 = Unbundle By Name(w462) -> ("Cond"=w463:bool)
    n287 = Unbundle By Name(w435) -> ("Turb"=w437:bool)
    n288 = Unbundle By Name(w446) -> ("Turb"=w445:bool)
    n289 = Unbundle By Name(w422) -> ("ORP"=w424:bool)
    n290 = Unbundle By Name(w433) -> ("ORP"=w432:bool)
    n291 = Unbundle By Name(w421) -> ("叶绿素a"=w419:bool)
    n292 = Unbundle By Name(w410) -> ("叶绿素a"=w411:bool)
    n293 = Unbundle By Name(w396) -> ("藻密度"=w398:bool)
    n294 = Unbundle By Name(w407) -> ("藻密度"=w406:bool)
    n295 = Unbundle By Name(w383) -> ("COD"=w382:bool)
    n296 = Unbundle By Name(w376) -> ("cod"=w377:bool)
    n297 = Unbundle By Name(w369) -> ("DO2"=w367:bool)
    n298 = Unbundle By Name(w358) -> ("DO2"=w359:bool)
    n299 = Boolean Array To Number(Boolean array=w479) -> (number=w478:u32)
    n300 = Boolean Array To Number(Boolean array=w481) -> (number=w482:u32)
    n301 = Boolean Array To Number(Boolean array=w453) -> (number=w452:u32)
    n302 = Boolean Array To Number(Boolean array=w455) -> (number=w456:u32)
    n303 = Boolean Array To Number(Boolean array=w468) -> (number=w469:u32)
    n304 = Boolean Array To Number(Boolean array=w466) -> (number=w465:u32)
    n305 = Boolean Array To Number(Boolean array=w440) -> (number=w439:u32)
    n306 = Boolean Array To Number(Boolean array=w442) -> (number=w443:u32)
    n307 = Boolean Array To Number(Boolean array=w427) -> (number=w426:u32)
    n308 = Boolean Array To Number(Boolean array=w429) -> (number=w430:u32)
    n309 = Boolean Array To Number(Boolean array=w416) -> (number=w417:u32)
    n310 = Boolean Array To Number(Boolean array=w414) -> (number=w413:u32)
    n311 = Boolean Array To Number(Boolean array=w401) -> (number=w400:u32)
    n312 = Boolean Array To Number(Boolean array=w403) -> (number=w404:u32)
    n313 = Boolean Array To Number(Boolean array=w379) -> (number=w380:u32)
    n314 = Boolean Array To Number(Boolean array=w375) -> (number=w374:u32)
    n315 = Boolean Array To Number(Boolean array=w364) -> (number=w365:u32)
    n316 = Boolean Array To Number(Boolean array=w362) -> (number=w361:u32)
    n317 = Equal To 0?(x=w478) -> (x = 0?=w477:bool)
    n318 = Equal To 0?(x=w482) -> (x = 0?=w483:bool)
    n319 = Equal To 0?(x=w452) -> (x = 0?=w451:bool)
    n320 = Equal To 0?(x=w456) -> (x = 0?=w457:bool)
    n321 = Equal To 0?(x=w469) -> (x = 0?=w470:bool)
    n322 = Equal To 0?(x=w465) -> (x = 0?=w464:bool)
    n323 = Equal To 0?(x=w439) -> (x = 0?=w438:bool)
    n324 = Equal To 0?(x=w443) -> (x = 0?=w444:bool)
    n325 = Equal To 0?(x=w426) -> (x = 0?=w425:bool)
    n326 = Equal To 0?(x=w430) -> (x = 0?=w431:bool)
    n327 = Equal To 0?(x=w417) -> (x = 0?=w418:bool)
    n328 = Equal To 0?(x=w413) -> (x = 0?=w412:bool)
    n329 = Equal To 0?(x=w400) -> (x = 0?=w399:bool)
    n330 = Equal To 0?(x=w404) -> (x = 0?=w405:bool)
    n331 = Equal To 0?(x=w380) -> (x = 0?=w381:bool)
    n332 = Equal To 0?(x=w374) -> (x = 0?=w378:bool)
    n333 = Equal To 0?(x=w365) -> (x = 0?=w366:bool)
    n334 = Equal To 0?(x=w361) -> (x = 0?=w360:bool)
    n335 = Or(x=w476, y=w477) -> (x .or. y?=w475:bool)
    n336 = Or(x=w484, y=w483) -> (x .or. y?=w486:bool)
    n337 = Or(x=w450, y=w451) -> (x .or. y?=w449:bool)
    n338 = Or(x=w458, y=w457) -> (x .or. y?=w460:bool)
    n339 = Or(x=w471, y=w470) -> (x .or. y?=w472:bool)
    n340 = Or(x=w463, y=w464) -> (x .or. y?=w461:bool)
    n341 = Or(x=w437, y=w438) -> (x .or. y?=w436:bool)
    n342 = Or(x=w445, y=w444) -> (x .or. y?=w447:bool)
    n343 = Or(x=w424, y=w425) -> (x .or. y?=w423:bool)
    n344 = Or(x=w432, y=w431) -> (x .or. y?=w434:bool)
    n345 = Or(x=w419, y=w418) -> (x .or. y?=w420:bool)
    n346 = Or(x=w411, y=w412) -> (x .or. y?=w409:bool)
    n347 = Or(x=w398, y=w399) -> (x .or. y?=w397:bool)
    n348 = Or(x=w406, y=w405) -> (x .or. y?=w408:bool)
    n349 = Or(x=w382, y=w381) -> (x .or. y?=w373:bool)
    n350 = Or(x=w377, y=w378) -> (x .or. y?=w372:bool)
    n351 = Or(x=w367, y=w366) -> (x .or. y?=w368:bool)
    n352 = Or(x=w359, y=w360) -> (x .or. y?=w357:bool)
    n353 = global read "断电保存变量.vi" "pH"() -> (w480:bool)
    n354 = global read "断电保存变量.vi" "DO"() -> (w454:bool)
    n355 = global read "断电保存变量.vi" "Cond"() -> (w467:bool)
    n356 = global read "断电保存变量.vi" "Turb"() -> (w441:bool)
    n357 = global read "断电保存变量.vi" "orp"() -> (w428:bool)
    n358 = global read "断电保存变量.vi" "叶绿素a启用"() -> (w415:bool)
    n359 = global read "断电保存变量.vi" "藻密度"() -> (w402:bool)
    n360 = global read "断电保存变量.vi" "COD"() -> (w384:bool)
    n361 = global read "断电保存变量.vi" "DO 2"() -> (w363:bool)
    n362 = Compound Arithmetic op=AND ("复合运算")(w480, w475, w486) -> (w395:bool)
    n363 = Compound Arithmetic op=AND ("复合运算")(w454, w449, w460) -> (w370:bool)
    n364 = Compound Arithmetic op=AND ("复合运算")(w467, w472, w461) -> (w394:bool)
    n365 = Compound Arithmetic op=AND ("复合运算")(w441, w436, w447) -> (w393:bool)
    n366 = Compound Arithmetic op=AND ("复合运算")(w428, w423, w434) -> (w392:bool)
    n367 = Compound Arithmetic op=AND ("复合运算")(w415, w420, w409) -> (w391:bool)
    n368 = Compound Arithmetic op=AND ("复合运算")(w402, w397, w408) -> (w390:bool)
    n369 = Compound Arithmetic op=AND ("复合运算")(w384, w373, w372) -> (w371:bool)
    n370 = Compound Arithmetic op=AND ("复合运算")(w363, w368, w357) -> (w356:bool)
    n371 = Build Array(w395, w370, w394, w393, w392, w391, w390, w371, w356) -> (w389:bool[])
    n372 = for {
      tunnel: w389 -> [w494] mode=indexing
      tunnel: w388 -> [w495] mode=indexing
      tunnel: [w495] -> w387 mode=indexing if=w494
      tunnel: [w493] -> w355
      i -> [w493]
    }
    n373 = Less Or Equal?(x=w355, y=1) -> (x <= y?=w353:bool)
    n374 = Select(t=u32 2000 ("等待时间（毫秒）"), s=w353, f=u32 1000 ("等待时间（毫秒）")) -> (s? t:f=w350:u32)
    n375 = Wait (ms)(milliseconds to wait=w350) -> (millisecond timer value=w349:u32)
    n376 = Get Queue Status(queue=w488) -> (queue out=w386:refnum<queue>, # elements in queue=w385:i32)  [unwired: 2 in, 6 out]
    n377 = case shown="0" w385 {
      tunnel: w387 -> [_ w490]
      tunnel: w386 -> [_ w489]
      tunnel: w349 -> [_ _]
      frame Default {
      }
      frame 0 {
        n378 = for {
          tunnel: w489 -> [w492]
          tunnel: w490 -> [w491] mode=indexing
          n379 = Enqueue Element(queue=w492, element=w491) -> ()  [unwired: 2 in, 3 out]
        }
      }
    }
  }
